vi "RPI2 Check UART Console.vi"(8 "Error In":errorcluster, 10 "Warnings":T1[](array[typedef]), 11 "Install LV Data":T2={"SSH Session"=refnum, "Status Log"="", "Detailed Log"="", "Credentials"={"Hostname or IP"="192.168.7.2", "Username"="root", "Password"=""}, "Target Info"={"OS Version"="", "CPU"="", "Systemd Version"="", "Internet Access"=FALSE, "Device Type"="", "LV Installed Ver"="", "LV Available Ver"="", "LV Upgrade Available"=FALSE, "Hostname"="", "NIC Info"=[]}, "Reboot Required?"=FALSE}) -> (0 "Error Out":errorcluster, 2 "Warnings":T1[](array[typedef]), 3 "Install LV Data":T2={"SSH Session"=refnum, "Status Log"="", "Detailed Log"="", "Credentials"={"Hostname or IP"="192.168.7.2", "Username"="root", "Password"=""}, "Target Info"={"OS Version"="", "CPU"="", "Systemd Version"="", "Internet Access"=FALSE, "Device Type"="", "LV Installed Ver"="", "LV Available Ver"="", "LV Upgrade Available"=FALSE, "Hostname"="", "NIC Info"=[]}, "Reboot Required?"=FALSE})   [LabVIEW 2020, in "LMH-LINX.lvlib"]
uses:
  LMH-LINX.lvlib
  Install LV Data.ctl
  Target Info.ctl
  NIC Info.ctl
  NIC Mode.ctl
  Target Compatibility Warnings.ctl
  RPI2 Enable UART.vi
  <vilib>/regexp/Match Regular Expression.xnode
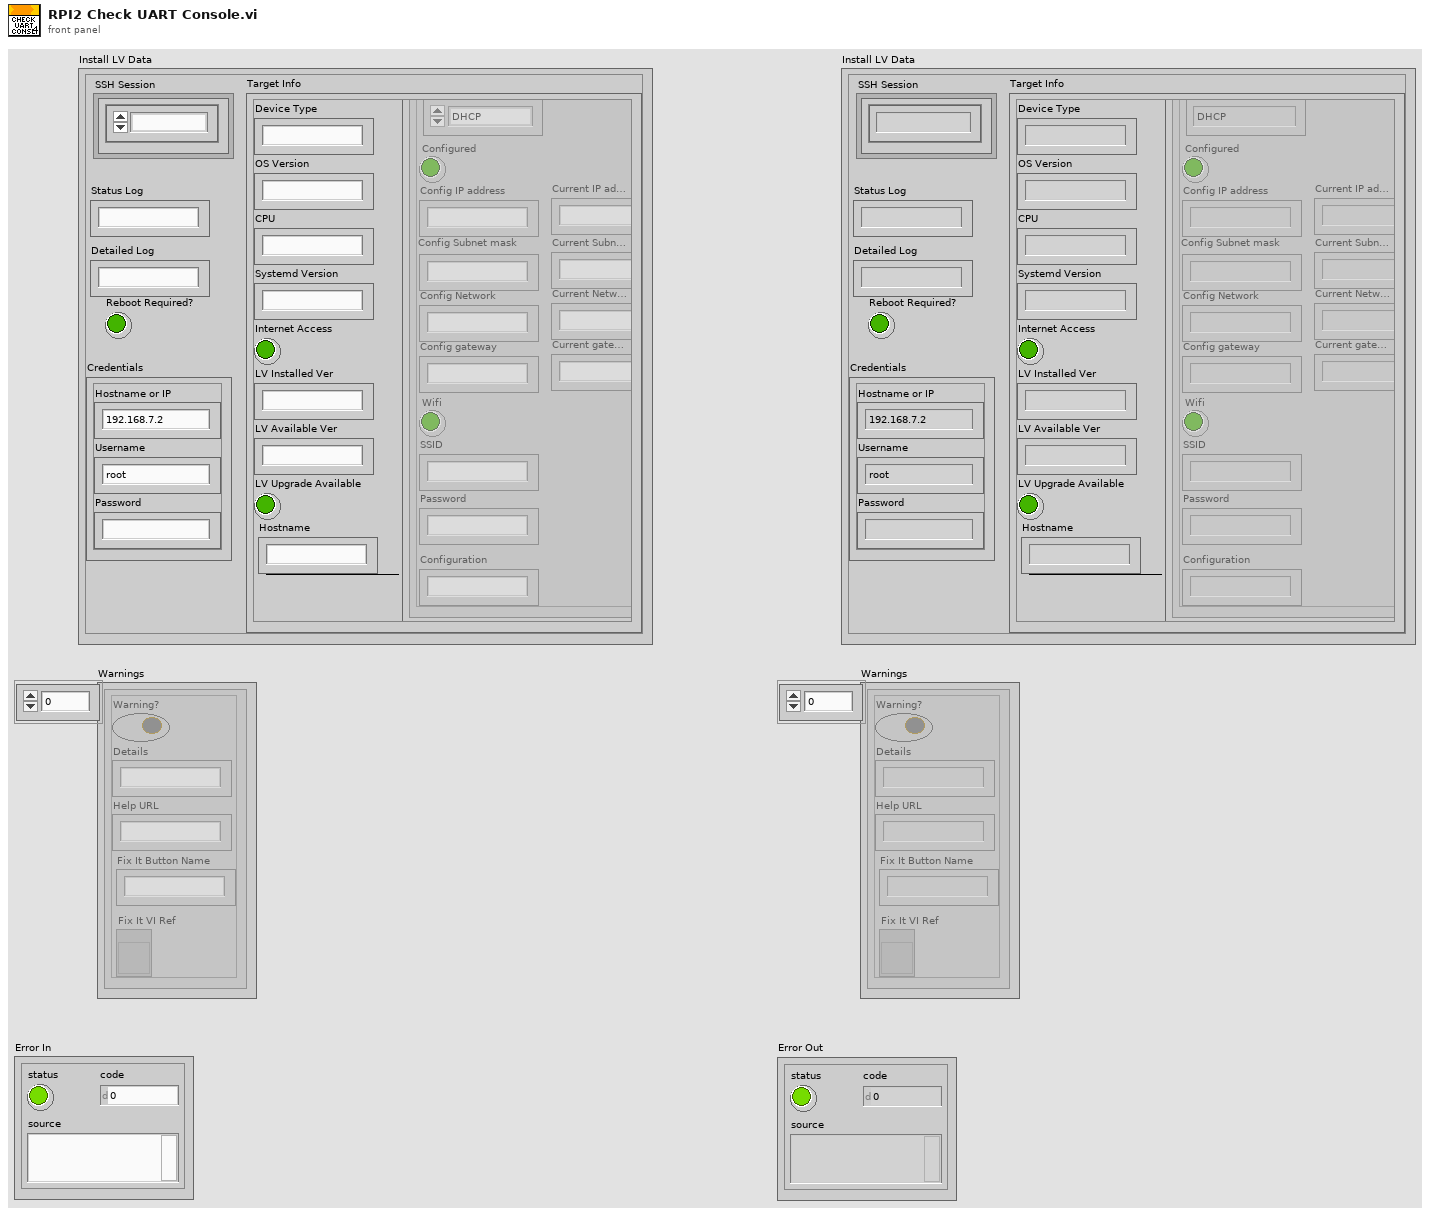
[diagram p1: front panel]
types:
  T1 = typedef "LMH-LINX.lvlib/Target Compatibility Warnings.ctl" = cluster{"Warning?":bool, "Details":string, "Help URL":string, "Fix It Button Name":string, "Fix It VI Ref":refnum<vi>}
  T2 = typedef "LMH-LINX.lvlib/Install LV Data.ctl" = cluster{"SSH Session":refnum<k1>, "Status Log":string, "Detailed Log":string, "Credentials":cluster{"Hostname or IP":string, "Username":string, "Password":string}, "Target Info":T3, "Reboot Required?":bool}
  T3 = typedef "LMH-LINX.lvlib/Target Info.ctl" = cluster{"OS Version":string, "CPU":string, "Systemd Version":string, "Internet Access":bool, "Device Type":string, "LV Installed Ver":string, "LV Available Ver":string, "LV Upgrade Available":bool, "Hostname":string, "NIC Info":T4[]}
  T4 = typedef "LMH-LINX.lvlib/NIC Info.ctl" = cluster{"Name":string, "NIC Mode":T5, "Configured":bool, "Config IP address":string, "Config Subnet mask":string, "Config Network":string, "Config gateway":string, "Wifi":bool, "SSID":string, "Password":string, "Configuration":string, "Current IP address":string, "Current Subnet mask":string, "Current gateway":string, "Current Network":string}
  T5 = typedef "LMH-LINX.lvlib/NIC Mode.ctl" = enum16{"DHCP", "Static", "Loopback"}
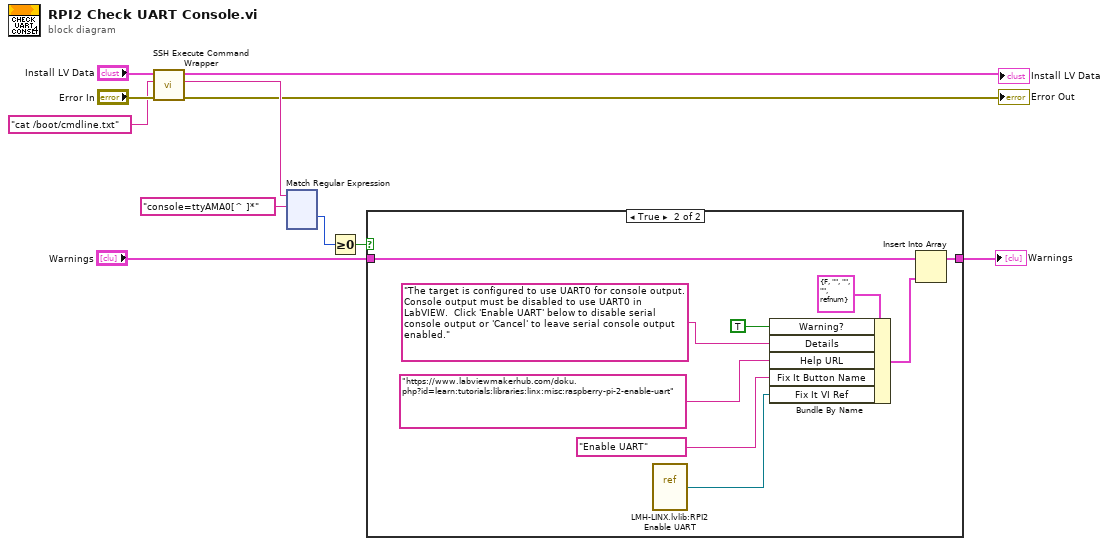
[diagram p0: block diagram]
diagram:
  n1 = call "SSH Execute Command Wrapper.vi"("Error In"="Error In", "Command"="cat /boot/cmdline.txt", "Install LV Data in"="Install LV Data") -> ("Error Out"=→"Error Out":errorcluster, "Std Out"=w4:string, "Install LV Data out"=→"Install LV Data":T2)  [unwired: 6 in]
  n2 = xnode "Match Regular Expression"("input string"=w4, "regular expression"="console=ttyAMA0[^ ]*" ("search string/char (-)")) -> ("offset past match"=w3:i32)  [unwired: 4 in, 4 out]
  n3 = Greater Or Equal To 0?(x=w3) -> (x >= 0?=w2:bool)
  n4 = case shown="True" w2 {
    tunnel: "Warnings" -> [w12 w21]
    tunnel: [w12 w20] -> w10
    frame False {
    }
    frame True {
      n5 = vi-ref "LMH-LINX.lvlib:RPI2 Enable UART.vi"() -> (w14:refnum<vi>)
      n6 = Bundle By Name(cluster=T1 {"Warning?"=FALSE, "Details"="", "Help URL"="", "Fix It Button Name"="", "Fix It VI Ref"=refnum} ("Target Compatibility Warnings"), "Warning?"=TRUE ("Can Continue?"), "Details"="The target is configured to use UART0 for console output.  Console output must be disabled to use UART0 in LabVIEW.  Click 'Enable UART' below to disable serial console output or 'Cancel' to leave serial console output enabled." ("string"), "Help URL"="https://www.labviewmakerhub.com/doku.php?id=learn:tutorials:libraries:linx:misc:raspberry-pi-2-enable-uart" ("string"), "Fix It Button Name"="Enable UART" ("string"), "Fix It VI Ref"=w14) -> (w17:T1)
      n7 = Insert Into Array(array=w21, new element=w17) -> (w20:T1[])  [unwired: 1 in]
    }
  }
  "Warnings" <- w10
